vi "Append.vi"() -> ()   [LabVIEW 2013]
uses:
  Tools/Line.ctl
  Global.vi
panel:
  in  "SEQ":T1[](array[typedef])
  in  "Append":bool
  out "#":i32
  in  "Output":T1[](array[typedef])
  in  "Save":path
  in  "Stop Button":bool
  in  "Open":path
  in  "Save Button":bool
  in  "Load Button":bool
  # "Append"
  # "append SEQ to output"
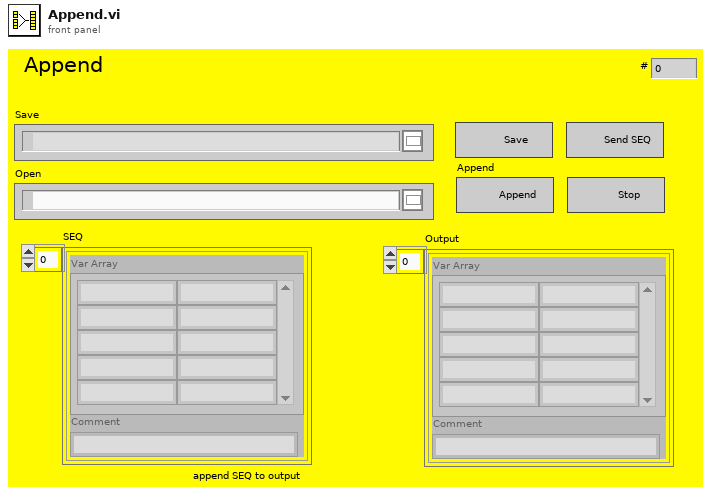
[diagram p1: front panel]
types:
  T1 = typedef "Line.ctl" = cluster{"Var Array":string[][], "Comment":string}
  T2 = enum16{"Left Button", "Center Button", "Right Button", "Window Close"}
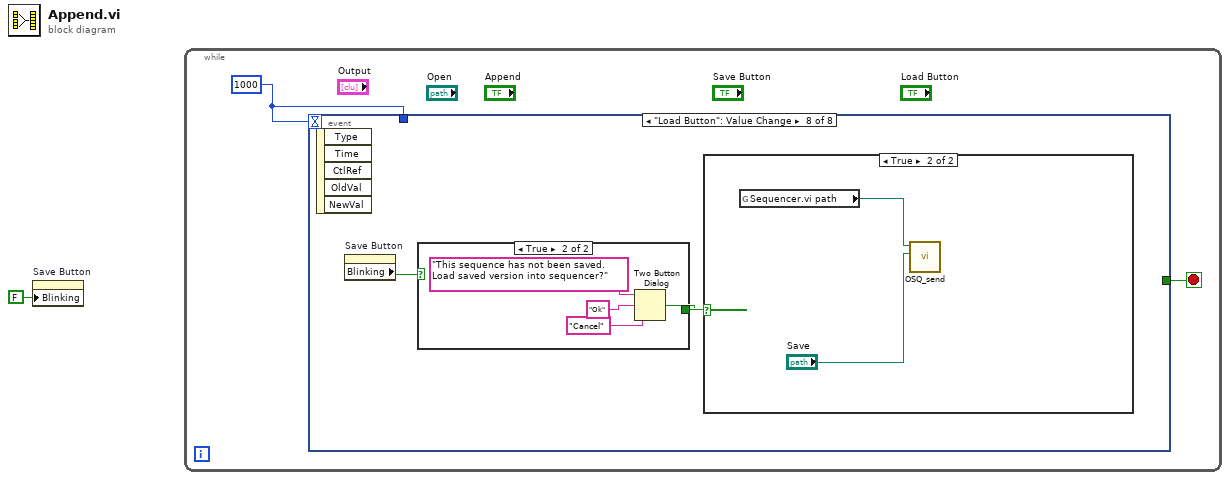
[diagram p0: block diagram]
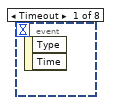
[diagram p2: hidden frame]
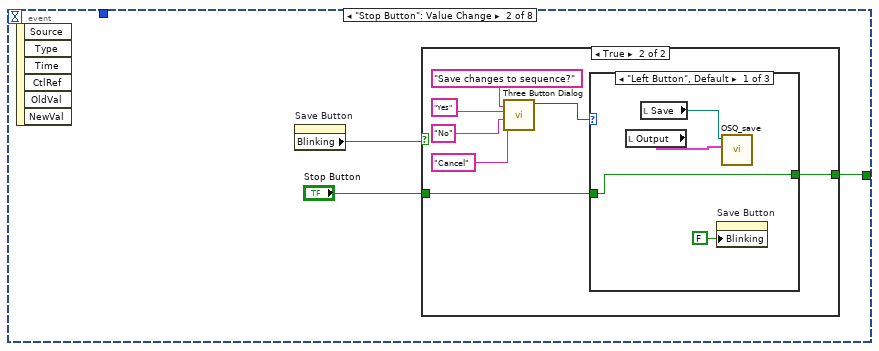
[diagram p3: hidden frame]
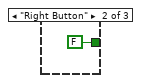
[diagram p5: hidden frame]
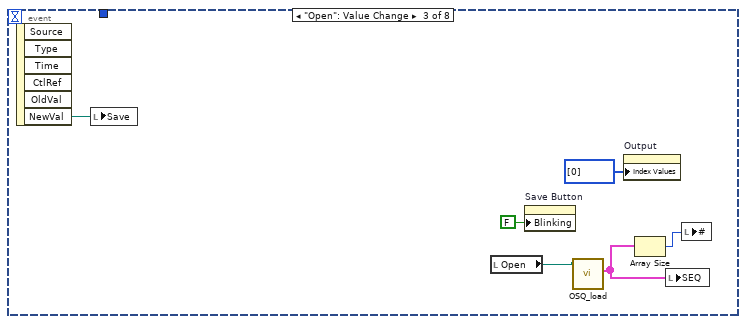
[diagram p7: hidden frame]
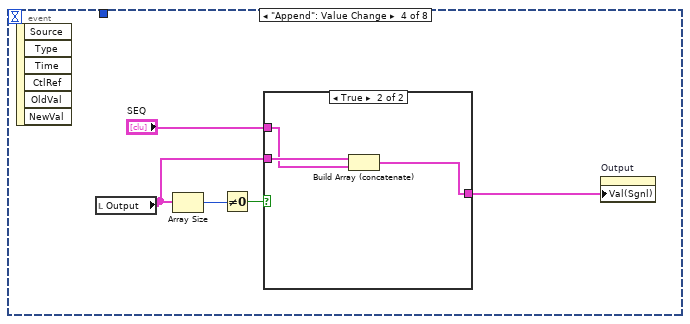
[diagram p8: hidden frame]
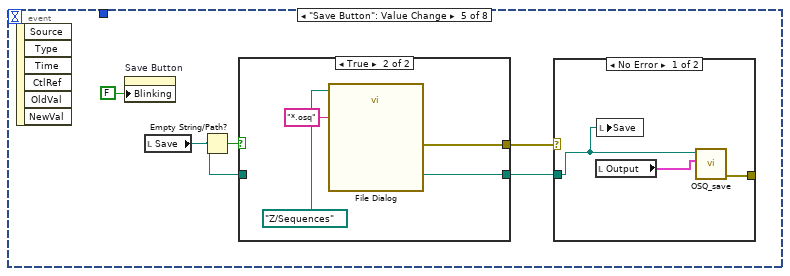
[diagram p10: hidden frame]
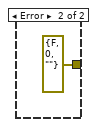
[diagram p11: hidden frame]
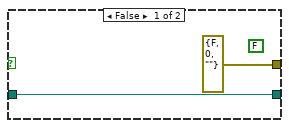
[diagram p12: hidden frame]
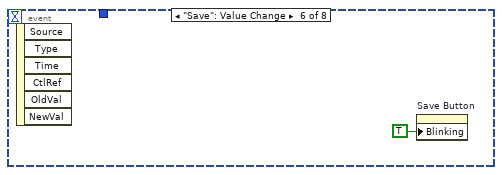
[diagram p13: hidden frame]
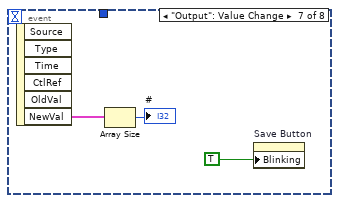
[diagram p14: hidden frame]
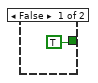
[diagram p16: hidden frame]
diagram:
  n1 = property on="Save Button" class="Bool"("Blinking"=FALSE) -> ()  [unwired: 2 in, 2 out]
  n2 = while {
    stop <- w3 stop-if-true
    w2 = 1000
    n3 = event shown="[7] \"Load Button\": Value Change" {
      selector: _ -> [_ _ _ _ _ _ _ _]
      dyn-events: _ -> [_ _ _ _ _ _ _ _]
      timeout: w2 -> [_ _ _ _ _ _ _ _]
      tunnel: [_ w6 _ _ _ _ _ _] -> w3
      tunnel: w2 -> [_ _ _ _ _ _ _ _]
      event Timeout {
        n4 = event-data() -> ()  [unwired: 1 in, 2 out]
      }
      event "Stop Button": Value Change {
        n5 = event-data() -> ()  [unwired: 1 in, 6 out]
        n6 = property on="Save Button" class="Bool"() -> ("Blinking"=w5:bool)  [unwired: 2 in, 2 out]
        n7 = case shown="True" w5 {
          tunnel: [w7 w8] -> w6
          tunnel: "Stop Button" -> [w7 w9]
          frame False {
          }
          frame True {
            n8 = call <vilib>:"Three Button Dialog.vi"("Right Button Text (\"Cancel\")"="Cancel" ("Right Button Text (\"Cancel\")"), "Center Button Text (\"No\")"="No" ("F button name (\"Cancel\")"), "Left Button Text (\"Yes\")"="Yes" ("T button name (\"OK\")"), "message"="Save changes to sequence?") -> ("Which Button?"=w10:T2)  [unwired: 7 in]
            n9 = case shown="\"Left Button\", Default" w10 {
              tunnel: w9 -> [w18 _ w20]
              tunnel: [w18 FALSE ("Stop Button") w20] -> w8
              frame "Left Button", Default {
                n10 = local read "Output"() -> (w15:T1[])
                n11 = local read "Save"() -> (w17:path)
                n12 = property on="Save Button" class="Bool"("Blinking"=FALSE) -> ()  [unwired: 2 in, 2 out]
                n13 = call "OSQ_save.vi"("SEQs"=w15, "Save"=w17) -> ()  [unwired: 8 in, 2 out]
              }
              frame "Right Button" {
              }
              frame "Center Button" {
              }
            }
          }
        }
      }
      event "Open": Value Change {
        n14 = event-data() -> ("NewVal"=w26:path)  [unwired: 1 in, 5 out]
        n15 = local write "Save"(w26) -> ()
        n16 = local read "Open"() -> (w24:path)
        n17 = property on="Save Button" class="Bool"("Blinking"=FALSE) -> ()  [unwired: 2 in, 2 out]
        n18 = call "OSQ_load.vi"("Open"=w24) -> ("SEQs"=w22:T1[])  [unwired: 7 in, 3 out]
        n19 = property on="Output" class="Arr (strict)"("Index Values"=u32[] [0]) -> ()  [unwired: 2 in, 2 out]
        n20 = Array Size(array=w22) -> (size(s)=w21:i32)
        n21 = local write "SEQ"(w22) -> ()
        n22 = local write "#"(w21) -> ()
      }
      event "Append": Value Change {
        n23 = event-data() -> ()  [unwired: 1 in, 6 out]
        n24 = local read "Output"() -> (w27:T1[])
        n25 = Array Size(array=w27) -> (size(s)=w31:i32)
        n26 = Not Equal To 0?(x=w31) -> (x != 0?=w30:bool)
        n27 = case shown="True" w30 {
          tunnel: "SEQ" -> [w32 w34]
          tunnel: [w32 w33] -> w28
          tunnel: w27 -> [_ w35]
          frame False {
          }
          frame True {
            n28 = Build Array (concatenate)(w35, w34) -> (w33:T1[])
          }
        }
        n29 = property on="Output" class="Arr (strict)"("Val(Sgnl)"=w28) -> ()  [unwired: 2 in, 2 out]
      }
      event "Save Button": Value Change {
        n30 = event-data() -> ()  [unwired: 1 in, 6 out]
        n31 = property on="Save Button" class="Bool"("Blinking"=FALSE) -> ()  [unwired: 2 in, 2 out]
        n32 = local read "Save"() -> (w38:path)
        n33 = Empty String/Path?(string/path=w38) -> (empty?=w39:bool)
        n34 = case shown="True" w39 {
          tunnel: [w46 w50] -> w37
          tunnel: w38 -> [w46 _]
          tunnel: [errorcluster {"status"=FALSE, "code"=0, "source"=""} ("error out") w47] -> w36
          frame False {
            (unwired) FALSE ("cancelled")
          }
          frame True {
            n35 = call "File Dialog"("start path"=path "Z:/Sequences", "pattern (all files)"="*.osq") -> ("selected path"=w50:path, "error out"=w47:errorcluster)  [unwired: 10 in, 2 out]
          }
        }
        n36 = case shown="No Error" w36 {
          tunnel: w37 -> [w42 _]
          tunnel: [w41 errorcluster {"status"=FALSE, "code"=0, "source"=""} ("error out")] -> _
          frame No Error {
            n37 = local read "Output"() -> (w43:T1[])
            n38 = local write "Save"(w42) -> ()
            n39 = call "OSQ_save.vi"("SEQs"=w43, "Save"=w42) -> ("error out"=w41:errorcluster)  [unwired: 8 in, 1 out]
          }
          frame Error {
          }
        }
      }
      event "Save": Value Change {
        n40 = event-data() -> ()  [unwired: 1 in, 6 out]
        n41 = property on="Save Button" class="Bool"("Blinking"=TRUE) -> ()  [unwired: 2 in, 2 out]
      }
      event "Output": Value Change {
        n42 = event-data() -> ("NewVal"=w53:T1[])  [unwired: 1 in, 5 out]
        n43 = Array Size(array=w53) -> (size(s)=→"#":i32)
        n44 = property on="Save Button" class="Bool"("Blinking"=TRUE) -> ()  [unwired: 2 in, 2 out]
      }
      event "Load Button": Value Change {
        n45 = event-data() -> ()  [unwired: 1 in, 5 out]
        n46 = property on="Save Button" class="Bool"() -> ("Blinking"=w56:bool)  [unwired: 2 in, 2 out]
        n47 = case shown="True" w56 {
          tunnel: [TRUE w60] -> w55
          frame False {
          }
          frame True {
            n48 = Two Button Dialog(message="This sequence has not been saved.  Load saved version into sequencer?", 1:"Cancel" ("F button name (\"Cancel\")"), 2:"Ok" ("T button name (\"OK\")")) -> (T button?=w60:bool)
          }
        }
        n49 = case shown="True" w55 {
          frame False {
          }
          frame True {
            n50 = global read "Global.vi" "Sequencer.vi path"() -> (w58:path)
            n51 = call "OSQ_send.vi"("Sequence File"="Save", "vi path"=w58) -> ()  [unwired: 10 in]
          }
        }
      }
    }
  }
